vi "Real SVD Decomposition.vi"(9 "SVD option":T2 items=["Thin", "Full"], 10 "singular values only?":bool, 11 "A":T1) -> (0 "error":i32, 1 "Matrix V":T1, 2 "Matrix S":T1, 3 "Matrix U":T1, 5 "Vector S":dbl[](array[numeric]))   [LabVIEW 2024, in "NI_AALPro.lvlib"]
doc: "<p>Computes the singular value decomposition (SVD) of the <em>m</em> <span class=\"U+215\">x</span> <em>n</em> matrix <strong>A</strong>. Wire data to the <strong>A</strong> input to determine the polymorphic instance to use or <a href=\"nihelplauncher://docs/csh?context=lvcore_lvhowto_selectingdefaultinstpolyvi\">manually select</a> the instance.\n</p>"
uses:
  NI_AALPro.lvlib
  RealMatrix.ctl
  SVD Option.ctl
  <resource>/lvanlys.dll
  NI_Matrix.lvlib
panel:
  # "SVD Decomposition"
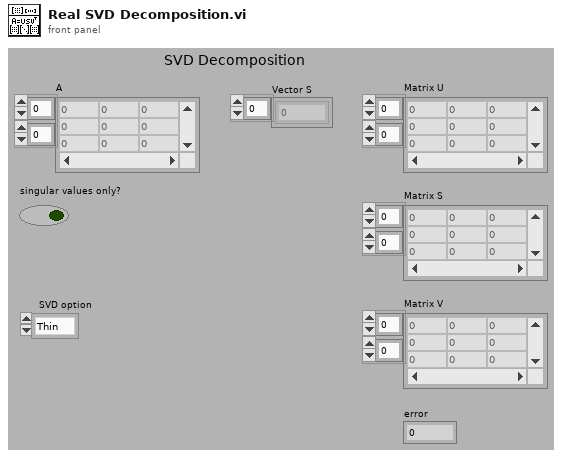
[diagram p1: front panel]
types:
  T1 = typedef "NI_Matrix.lvlib/RealMatrix.ctl" = dbl[][]
  T2 = typedef "NI_AALPro.lvlib/SVD Option.ctl" = u16
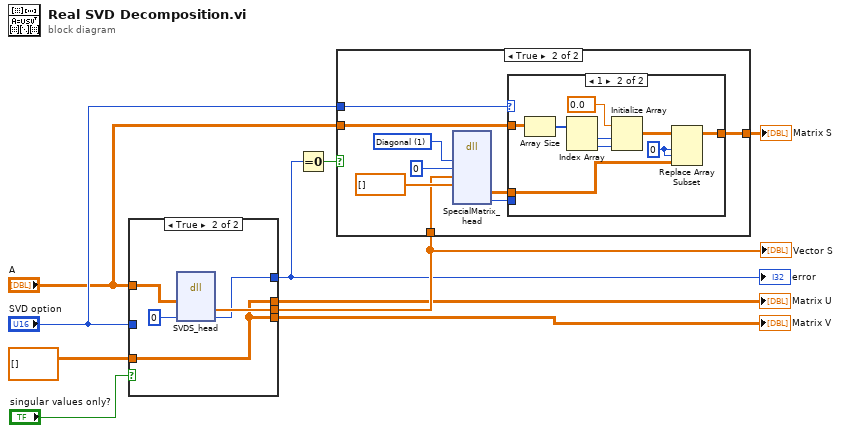
[diagram p0: block diagram]
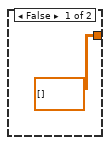
[diagram p2: hidden frame]
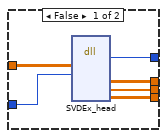
[diagram p4: hidden frame]
diagram:
  n1 = case shown="True" "singular values only?" {
    tunnel: [w13 w17] -> w5
    tunnel: [w16 w18] -> w2
    tunnel: "SVD option" -> [w15 _]
    tunnel: [w12 w19] -> w9
    tunnel: "A" -> [w14 w21]
    tunnel: [w11 w17] -> w6
    tunnel: dbl[][] [] ("V") -> [_ w17]
    frame False {
      n2 = dll-call lib="C:/Program Files (x86)/National Instruments/LabVIEW 2024/resource/lvanlys.*" fn="SVDEx_head"("aH"=w14, "flag"=w15) -> ("return type"=w16:i32, "uH"=w13:dbl[][], "sH"=w12:dbl[], "vH"=w11:dbl[][])  [unwired: 8 in, 2 out]
    }
    frame True {
      n3 = dll-call lib="C:/Program Files (x86)/National Instruments/LabVIEW 2024/resource/lvanlys.*" fn="SVDS_head"("aH"=w21, "dsperr"=0 ("input param")) -> ("wH"=w19:dbl[], "dsperr"=w18:i32)  [unwired: 6 in, 2 out]
    }
  }
  "Matrix U" <- w5
  "Matrix V" <- w6
  "error" <- w2
  "Vector S" <- w9
  n4 = Equal To 0?(x=w2) -> (x = 0?=w3:bool)
  n5 = case shown="True" w3 {
    tunnel: "SVD option" -> [_ w31]
    tunnel: w9 -> [_ w25]
    tunnel: "A" -> [_ w30]
    tunnel: [dbl[][] [] ("Special Matrix") w29] -> w4
    frame False {
    }
    frame True {
      w28 = 1 items=["Identity", "Diagonal", "Toepliz", "Vandermonde", "Companion", "Hankel", "Hadamard", "Wilkinson", "Hilbert", "Inverse Hilbert", "Rosser", "Pascal"] ("matrix type")
      n6 = dll-call lib="C:/Program Files (x86)/National Instruments/LabVIEW 2024/resource/lvanlys.*" fn="SpecialMatrix_head"("mtype"=w28, "msize"=0 ("matrix size"), "v1H"=w25, "v2H"=dbl[] [] ("S")) -> ("aH"=w24:dbl[][], "dsperr"=w23:i32)  [unwired: 10 in, 2 out]
      n7 = case shown="1" w31 {
        tunnel: [w32 w33] -> w29
        tunnel: w24 -> [w32 w34]
        tunnel: w30 -> [_ w38]
        tunnel: w23 -> [_ _]
        frame 0, Default {
        }
        frame 1 {
          w35 = 0 ("index (row)")
          n8 = Array Size(array=w38) -> (size(s)=w37:i32[])
          n9 = Index Array(array=w37) -> (element #1=w40:i32, element #2=w39:i32)  [unwired: 2 in]
          n10 = Initialize Array(0.0 ("element"), w40, w39) -> (w36:dbl[][])
          n11 = Replace Array Subset(array=w36, new element=w34, index (row)=w35, index (col)=w35) -> (w33:dbl[][])
        }
      }
    }
  }
  "Matrix S" <- w4
